vi "ArrayFFT.vi"(3 "Period":u16, 5 "Array":fxp<+/-,16,4>[](array[numeric])) -> (1 "Max":fxp<+,16,4>)   [LabVIEW 2015]
uses:
  <vilib>/rvi/Analysis/measure/FFT/simModelSupport/niFPGA FFT Outside SCTL Sim Properties.ctl
  <vilib>/rvi/Analysis/measure/FFT/simModelSupport/niFPGA FFT Sim Types.ctl
  <vilib>/rvi/Analysis/measure/FFT/simModelSupport/niFpgaFFTSimArithmeticProperties.ctl
  <vilib>/rvi/Analysis/measure/FFT/simModelSupport/niFpgaFFTSimDfxp.ctl
  <vilib>/fxp/LVFixedPointQuantizationPolicyTypeDef.ctl
  <vilib>/rvi/Analysis/measure/FFT/simModelSupport/niFpgaFFTSimModelOutsideSCTLCore.vi
  <vilib>/rvi/Analysis/measure/FFT/XNode/niFpgaFFT.xnode
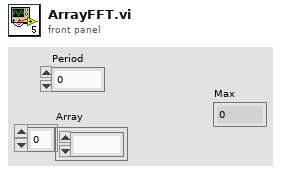
[diagram p1: front panel]
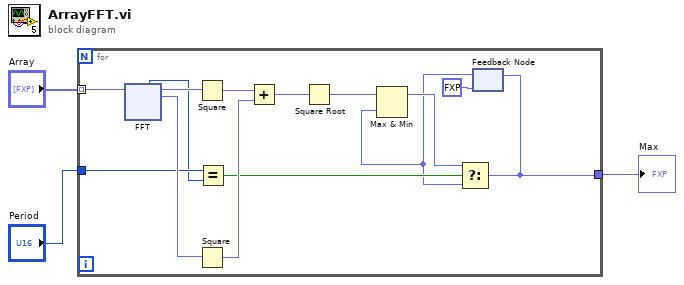
[diagram p0: block diagram]
diagram:
  n1 = for {
    tunnel: "Array" -> [w12] mode=indexing
    tunnel: "Period" -> [w11]
    tunnel: [w5] -> w1
    n2 = xnode "FFT"("real data in"=w12) -> ("data index"=w4:u16, "real data out"=w14:fxp<+/-,26,14>, "imaginary data out"=w13:fxp<+/-,26,14>)  [unwired: 2 in]
    n3 = Square(x=w14) -> (x^2=w15:fxp<+,51,27>)
    n4 = Square(x=w13) -> (x^2=w16:fxp<+,51,27>)
    n5 = Equal?(x=w11, y=w4) -> (x = y?=w8:bool)
    n6 = Add(x=w15, y=w16) -> (x+y=w17:fxp<+,52,28>)
    n7 = Square Root(x=w17) -> (sqrt(x)=w9:fxp<+,16,4>)
    n8 = feedback #1(fxp<+,16,4> 0.0) -> (w6:fxp<+,16,4>)
    n9 = Max & Min(x=w9, y=w6) -> (max(x,y)=w7:fxp<+,16,4>)  [unwired: 1 out]
    n10 = Select(t=w7, s=w8, f=w6) -> (s? t:f=w5:fxp<+,16,4>)
    n11 = feedback-in #1(w5) -> ()
  }
  "Max" <- w1
